vi "Reset Measurements.vi"   [LabVIEW 2012, in "NH Research Regenerative Test Series.lvlib"]
doc: "Resets measurements within instrument."
uses:
  <instrlib>/NH Research Regenerative Test Series/NH Research Regenerative Test Series.lvlib
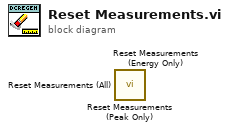
[diagram p0: block diagram]
diagram:
  n1 = call <instrlib>:"Reset Measurements (Peak Only).vi"() -> ()  [unwired: 14 in, 2 out]
  n2 = call <instrlib>:"Reset Measurements (Energy Only).vi"() -> ()  [unwired: 14 in, 2 out]
  n3 = call <instrlib>:"Reset Measurements (All).vi"() -> ()  [unwired: 14 in, 2 out]
